vi "Autonomous Independent.vi"   [LabVIEW 2012]
doc: "This VI is called when autonomous begins, and will automatically be terminated when autonomous ends. You can carry out timed or sensor driven robot movement independently without needing to return to the caller."
uses:
  <vilib>/Rock Robotics/WPI/Relay/WPI_RelayValue.ctl
  Robot Global Data.vi
types:
  T1 = typedef "WPI_EncoderDevRef.ctl" = cluster{"DevStatus":errorcluster, "EncoderIndex":T2, "CounterIndex":T3, "DistancePerCount":dbl, "Decoding Type":T4}
  T2 = typedef "FPGA_EncoderIdx.ctl" = enum8{"Enc 0", "Enc 1", "Enc 2", "Enc 3", "Invalid"}
  T3 = typedef "FPGA_CounterCtrSystemIndex.ctl" = enum8{"Ctr 0", "Ctr 1", "Ctr 2", "Ctr 3", "Ctr 4", "Ctr 5", "Ctr 6", "Ctr 7", "Invalid"}
  T4 = typedef "WPI_EncoderType.ctl" = enum16{"1x", "2x", "4x"}
  T5 = typedef "WPI_GyroDevRef.ctl" = cluster{"DevStatus":errorcluster, "Analog Module":T6, "Analog Channel":T7, "Offset":dbl, "Gain (VoltsPerDegree/Second)":dbl}
  T6 = typedef "FPGA_TypedefAnalogModule.ctl" = enum16{"Analog Module 1", "Analog Module 2"}
  T7 = typedef "FPGA_AIChannel.ctl" = enum8{"AI 1", "AI 2", "AI 3", "AI 4", "AI 5", "AI 6", "AI 7", "AI 8", "Invalid"}
  T8 = typedef "WPI_RelayValue.ctl" = enum16{"Off", "On", "Forward", "Reverse"}
  T9 = typedef "WPI_MotorControlDeviceRef.ctl" = cluster{"DeviceStatus":errorcluster, "Type":enum16{"PWM", "CAN"}, "PWM":cluster{"Digital Module":T10, "PWM Channel":T11, "DeadBand":T12}, "CAN":cluster{"Device Number":u8, "Control Mode":T13, "Semaphore":T14, "Max Vout":dbl}, "Invert":bool, "TransformRef":T15, "InvTransformRef":T15}
  T10 = typedef "FPGA_TypedefDigitalModule.ctl" = enum16{"Digital Module 1", "Digital Module 2"}
  T11 = typedef "FPGA_DIOPWMChannel.ctl" = enum8{"PWM 1", "PWM 2", "PWM 3", "PWM 4", "PWM 5", "PWM 6", "PWM 7", "PWM 8", "PWM 9", "PWM 10", "Invalid"}
  T12 = typedef "WPI_PWMDeadband.ctl" = cluster{"Name":string, "maxPositivePwm":i32, "minPositivePwm":i32, "centerPwm":i32, "maxNegativePwm":i32, "minNegativePwm":i32, "angularRange":u16}
  T13 = typedef "WPI_CANJaguar_ControlMode.ctl" = enum8{"Percent VBus", "Current", "Speed", "Position", "Voltage"}
  T14 = typedef "Semaphore RefNum" = refnum<k1>
  T15 = typedef "WPI_PWMTransform_ConPane.ctl" = refnum<vi>
  T16 = cluster{"Right Servo High":dbl, "Right Servo Mid":dbl, "Right Servo Low":dbl, "Left Servo High":dbl, "Left Servo Mid":dbl, "Left Servo Low":dbl}
  T17 = typedef "WPI_ServoDeviceRef.ctl" = cluster{"DeviceStatus":errorcluster, "Digital Module":T10, "PWM Channel":T11, "DeadBand":T12}
  T18 = typedef "WPI_RelayDevRef.ctl" = cluster{"DevStatus":errorcluster, "Relay Channel":T19, "Digital Module":T10, "Relay Direction":T20}
  T19 = typedef "FPGA_DIORelayChannel.ctl" = enum8{"Relay 1", "Relay 2", "Relay 3", "Relay 4", "Relay 5", "Relay 6", "Relay 7", "Relay 8", "Invalid"}
  T20 = typedef "WPI_RelayDirection.ctl" = enum16{"Both directions", "Forward only", "Reverse only"}
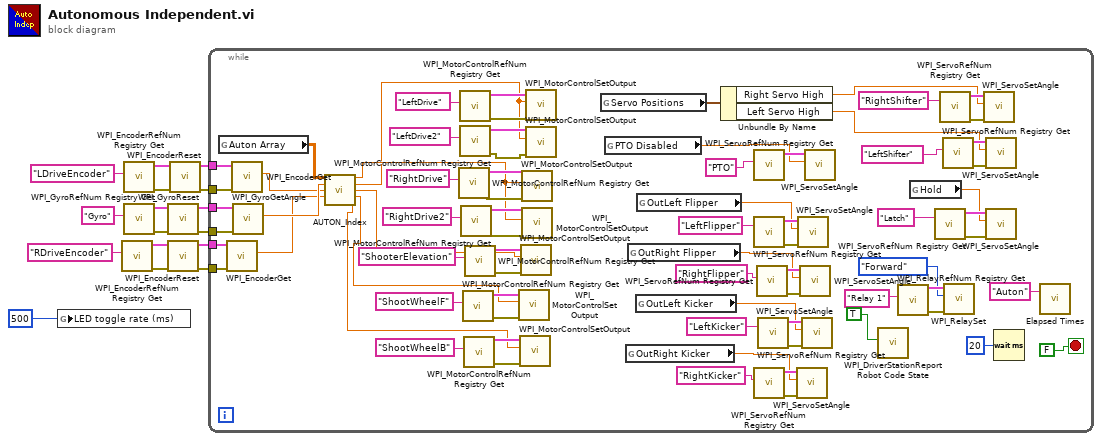
[diagram p0: block diagram]
diagram:
  n1 = global write "Robot Global Data.vi" "LED toggle rate (ms)"(u32 500 ("LED ms toggle rate")) -> ()
  n2 = call <vilib>:"WPI_EncoderRefNum Registry Get.vi"("refnum name"="RDriveEncoder") -> ("error out"=w3:errorcluster, "EncoderDevRef"=w5:T1)  [unwired: 9 in]
  n3 = call <vilib>:"WPI_EncoderRefNum Registry Get.vi"("refnum name"="LDriveEncoder") -> ("error out"=w9:errorcluster, "EncoderDevRef"=w8:T1)  [unwired: 9 in]
  n4 = call <vilib>:"WPI_GyroRefNum Registry Get.vi"("refnum name"="Gyro") -> ("error out"=w13:errorcluster, "GyroDevRef"=w14:T5)  [unwired: 9 in]
  n5 = call <vilib>:"WPI_GyroReset.vi"("error in (no error)"=w13, "GyroDevRef"=w14) -> ("error out"=w11:errorcluster, "GyroDevRef"=w12:T5)  [unwired: 8 in]
  n6 = call <vilib>:"WPI_EncoderReset.vi"("error in (no error)"=w3, "EncoderDevRef"=w5) -> ("error out"=w1:errorcluster, "EncoderDevRef"=w2:T1)  [unwired: 8 in]
  n7 = call <vilib>:"WPI_EncoderReset.vi"("error in (no error)"=w9, "EncoderDevRef"=w8) -> ("error out"=w6:errorcluster, "EncoderDevRef"=w7:T1)  [unwired: 8 in]
  n8 = while {
    tunnel: w12 -> [w88]
    tunnel: w11 -> [w87]
    tunnel: w7 -> [w86]
    tunnel: w6 -> [w85]
    tunnel: w2 -> [w77]
    tunnel: w1 -> [w76]
    stop <- FALSE stop-if-true
    n9 = global read "Robot Global Data.vi" "Auton Array"() -> (w78:dbl[][])
    n10 = call <vilib>:"WPI_EncoderGet.vi"("error in (no error)"=w76, "EncoderDevRef"=w77) -> ("Distance"=w75:dbl)  [unwired: 4 in, 5 out]
    n11 = call <vilib>:"WPI_EncoderGet.vi"("error in (no error)"=w85, "EncoderDevRef"=w86) -> ("Distance"=w84:dbl)  [unwired: 4 in, 5 out]
    n12 = call <vilib>:"WPI_GyroGetAngle.vi"("error in (no error)"=w87, "GyroDevRef"=w88) -> ("Angle"=w89:dbl)  [unwired: 6 in, 3 out]
    n13 = call "AUTON_Index.vi"("Auton Array"=w78, "MeasuredHeading"=w89, "LeftEncoder"=w84, "RightEncoder"=w75) -> ("Right Drive"=w31:dbl, "Left Drive"=w30:dbl, "Shooter Elevation"=w29:dbl, "Shooter Wheel F"=w18:dbl, "Shooter Wheel B"=w17:dbl)  [unwired: 7 in]
    n14 = call <vilib>:"WPI_MotorControlRefNum Registry Get.vi"("refnum name"="RightDrive") -> ("error out"=w32:errorcluster, "MotorControlDevRef"=w33:T9)  [unwired: 9 in]
    n15 = call <vilib>:"WPI_MotorControlRefNum Registry Get.vi"("refnum name"="LeftDrive") -> ("error out"=w38:errorcluster, "MotorControlDevRef"=w41:T9)  [unwired: 9 in]
    n16 = call <vilib>:"WPI_MotorControlRefNum Registry Get.vi"("refnum name"="LeftDrive2") -> ("error out"=w39:errorcluster, "MotorControlDevRef"=w40:T9)  [unwired: 9 in]
    n17 = call <vilib>:"WPI_MotorControlRefNum Registry Get.vi"("refnum name"="RightDrive2") -> ("error out"=w34:errorcluster, "MotorControlDevRef"=w35:T9)  [unwired: 9 in]
    n18 = call <vilib>:"WPI_MotorControlRefNum Registry Get.vi"("refnum name"="ShootWheelF") -> ("error out"=w24:errorcluster, "MotorControlDevRef"=w20:T9)  [unwired: 9 in]
    n19 = call <vilib>:"WPI_MotorControlRefNum Registry Get.vi"("refnum name"="ShootWheelB") -> ("error out"=w21:errorcluster, "MotorControlDevRef"=w19:T9)  [unwired: 9 in]
    n20 = call <vilib>:"WPI_MotorControlRefNum Registry Get.vi"("refnum name"="ShooterElevation") -> ("error out"=w36:errorcluster, "MotorControlDevRef"=w37:T9)  [unwired: 9 in]
    n21 = call <vilib>:"WPI_MotorControlSetOutput.vi"("error in (no error)"=w24, "Output"=w18, "MotorControlDevRef"=w20) -> ()  [unwired: 6 in, 3 out]
    n22 = call <vilib>:"WPI_MotorControlSetOutput.vi"("error in (no error)"=w21, "Output"=w17, "MotorControlDevRef"=w19) -> ()  [unwired: 6 in, 3 out]
    n23 = call <vilib>:"WPI_MotorControlSetOutput.vi"("error in (no error)"=w36, "Output"=w29, "MotorControlDevRef"=w37) -> ()  [unwired: 6 in, 3 out]
    n24 = call <vilib>:"WPI_MotorControlSetOutput.vi"("error in (no error)"=w32, "Output"=w31, "MotorControlDevRef"=w33) -> ()  [unwired: 6 in, 3 out]
    n25 = call <vilib>:"WPI_MotorControlSetOutput.vi"("error in (no error)"=w34, "Output"=w31, "MotorControlDevRef"=w35) -> ()  [unwired: 6 in, 3 out]
    n26 = call <vilib>:"WPI_MotorControlSetOutput.vi"("error in (no error)"=w38, "Output"=w30, "MotorControlDevRef"=w41) -> ()  [unwired: 6 in, 3 out]
    n27 = call <vilib>:"WPI_MotorControlSetOutput.vi"("error in (no error)"=w39, "Output"=w30, "MotorControlDevRef"=w40) -> ()  [unwired: 6 in, 3 out]
    n28 = global read "Robot Global Data.vi" "Servo Positions"() -> (w55:T16)
    n29 = global read "Robot Global Data.vi" "PTO Disabled"() -> (w44:dbl)
    n30 = global read "Robot Global Data.vi" "OutRight Kicker"() -> (w57:dbl)
    n31 = global read "Robot Global Data.vi" "OutRight Flipper"() -> (w61:dbl)
    n32 = global read "Robot Global Data.vi" "OutLeft Kicker"() -> (w56:dbl)
    n33 = global read "Robot Global Data.vi" "OutLeft Flipper"() -> (w59:dbl)
    n34 = Unbundle By Name(w55) -> ("Right Servo High"=w46:dbl, "Left Servo High"=w45:dbl)
    n35 = call <vilib>:"WPI_ServoRefNum Registry Get.vi"("refnum name"="PTO") -> ("ServoDeviceRef"=w48:T17)  [unwired: 9 in, 1 out]
    n36 = call <vilib>:"WPI_ServoRefNum Registry Get.vi"("refnum name"="LeftFlipper") -> ("error out"=w58:errorcluster, "ServoDeviceRef"=w60:T17)  [unwired: 9 in]
    n37 = call <vilib>:"WPI_ServoRefNum Registry Get.vi"("refnum name"="RightKicker") -> ("error out"=w69:errorcluster, "ServoDeviceRef"=w67:T17)  [unwired: 9 in]
    n38 = call <vilib>:"WPI_ServoRefNum Registry Get.vi"("refnum name"="RightFlipper") -> ("error out"=w71:errorcluster, "ServoDeviceRef"=w64:T17)  [unwired: 9 in]
    n39 = call <vilib>:"WPI_ServoRefNum Registry Get.vi"("refnum name"="LeftKicker") -> ("error out"=w62:errorcluster, "ServoDeviceRef"=w63:T17)  [unwired: 9 in]
    n40 = call <vilib>:"WPI_ServoSetAngle.vi"("error in (no error)"=w69, "Angle"=w57, "ServoDeviceRef"=w67) -> ()  [unwired: 7 in, 2 out]
    n41 = call <vilib>:"WPI_ServoSetAngle.vi"("error in (no error)"=w58, "Angle"=w59, "ServoDeviceRef"=w60) -> ()  [unwired: 7 in, 2 out]
    n42 = call <vilib>:"WPI_ServoSetAngle.vi"("error in (no error)"=w71, "Angle"=w61, "ServoDeviceRef"=w64) -> ()  [unwired: 7 in, 2 out]
    n43 = call <vilib>:"WPI_ServoSetAngle.vi"("error in (no error)"=w62, "Angle"=w56, "ServoDeviceRef"=w63) -> ()  [unwired: 7 in, 2 out]
    n44 = call <vilib>:"WPI_ServoSetAngle.vi"("Angle"=w44, "ServoDeviceRef"=w48) -> ()  [unwired: 8 in, 2 out]
    n45 = call <vilib>:"WPI_DriverStationReport Robot Code State.vi"("Autonomous"=TRUE) -> ()  [unwired: 10 in, 1 out]
    n46 = call <vilib>:"WPI_RelayRefNum Registry Get.vi"("refnum name"="Relay 1") -> ("error out"=w80:errorcluster, "RelayDevRef"=w82:T18)  [unwired: 9 in]
    n47 = global read "Robot Global Data.vi" "Hold"() -> (w25:dbl)
    n48 = call <vilib>:"WPI_ServoRefNum Registry Get.vi"("refnum name"="Latch") -> ("error out"=w26:errorcluster, "ServoDeviceRef"=w27:T17)  [unwired: 9 in]
    n49 = call <vilib>:"WPI_ServoRefNum Registry Get.vi"("refnum name"="RightShifter") -> ("error out"=w51:errorcluster, "ServoDeviceRef"=w52:T17)  [unwired: 9 in]
    n50 = call <vilib>:"WPI_ServoRefNum Registry Get.vi"("refnum name"="LeftShifter") -> ("error out"=w53:errorcluster, "ServoDeviceRef"=w54:T17)  [unwired: 9 in]
    n51 = call <vilib>:"WPI_RelaySet.vi"("error in (no error)"=w80, "RelayValue"=WPI_RelayValue."Forward", "RelayDevRef"=w82) -> ()  [unwired: 7 in, 2 out]
    n52 = call <vilib>:"WPI_ServoSetAngle.vi"("error in (no error)"=w51, "Angle"=w46, "ServoDeviceRef"=w52) -> ()  [unwired: 7 in, 2 out]
    n53 = call <vilib>:"WPI_ServoSetAngle.vi"("error in (no error)"=w53, "Angle"=w45, "ServoDeviceRef"=w54) -> ()  [unwired: 7 in, 2 out]
    n54 = call <vilib>:"WPI_ServoSetAngle.vi"("error in (no error)"=w26, "Angle"=w25, "ServoDeviceRef"=w27) -> ()  [unwired: 7 in, 2 out]
    n55 = Wait (ms)(milliseconds to wait=u32 20) -> ()  [unwired: 1 out]
    n56 = call "Elapsed Times.vi"("Call Name"="Auton") -> ()  [unwired: 2 in, 1 out]
  }
